vi "Print PDF.vi"(8 "error in (no error)":errorcluster, 11 "PDF Path":path) -> (0 "error out":errorcluster, 2 "Adobe Installed?":bool, 3 "Printed?":bool)   [LabVIEW 2011]
uses:
  <vilib>/registry/registry.llb/Registry RtKey.ctl
  OpenG EXT/file/file.llb/Strip Path Extension - Path__ogtk.vi
  <vilib>/registry/registry.llb/Read Registry Value Simple STR.vi
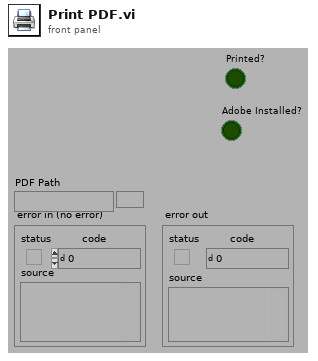
[diagram p1: front panel]
types:
  T1 = typedef "Registry RtKey.ctl" = enum32{"HKEY_CLASSES_ROOT", "HKEY_CURRENT_USER", "HKEY_LOCAL_MACHINE", "HKEY_USERS", "HKEY_PERFORMANCE_DATA", "HKEY_CURRENT_CONFIG", "HKEY_DYN_DATA"}
  T2 = typedef "Registry refnum.ctl" = refnum<k1>
  T3 = cluster{"numSubKeys":i32, "maxSubKeyLen":i32, "maxSubKeyClassLen":i32}
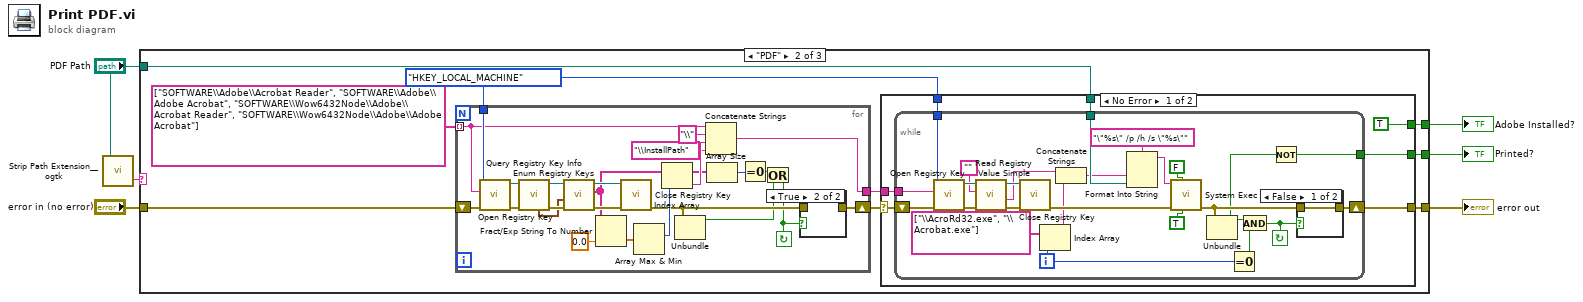
[diagram p0: block diagram]
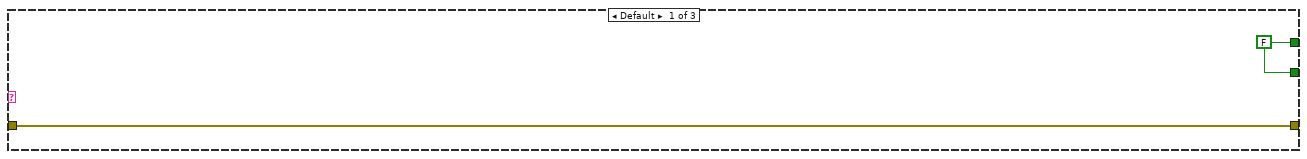
[diagram p2: hidden frame]
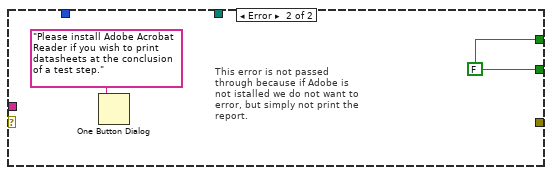
[diagram p5: hidden frame]
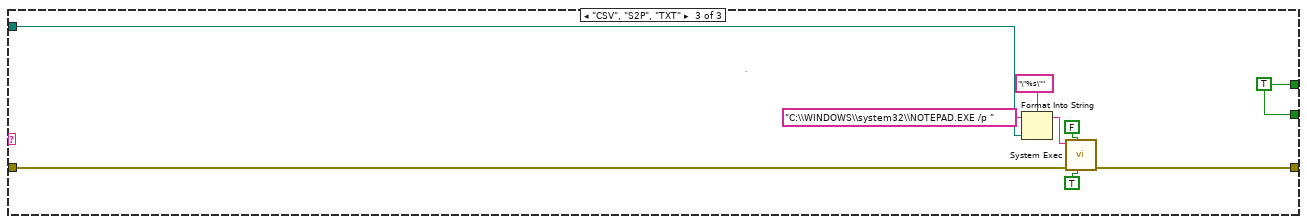
[diagram p6: hidden frame]
diagram:
  n1 = call-poly "Strip Path Extension__ogtk.vi"("path"="PDF Path") -> ("extension"=w1:string)  [unwired: 1 out]
  n2 = case shown="\"PDF\"" w1 {
    tunnel: "error in (no error)" -> [w7 w16 w81]
    tunnel: [w7 w14 w80] -> w5
    tunnel: [w8 w13 w78] -> w4
    tunnel: [w8 w12 w78] -> w3
    tunnel: "PDF Path" -> [_ w11 w86]
    frame Default {
      w8 = FALSE
    }
    frame "PDF" {
      w17 = Registry_RtKey."HKEY_LOCAL_MACHINE" ("root key (HKEY_LOCAL_MACHINE)")
      n3 = for {
        tunnel: [w28] -> w10
        tunnel: w17 -> [w27]
        shift-right: [w24] -> w15
        shift-left: w16 -> [w26]
        tunnel: string[] ["SOFTWARE\\Adobe\\Acrobat Reader", "SOFTWARE\\Adobe\\Adobe Acrobat", "SOFTWARE\\Wow6432Node\\Adobe\\Acrobat Reader", "SOFTWARE\\Wow6432Node\\Adobe\\Adobe Acrobat"] -> [w18] mode=indexing
        stop <- w19 continue-if-true
        n4 = call <vilib>:"Open Registry Key.vi"("error in (no error)"=w26, "subkey"=w18, "root key (HKEY_LOCAL_MACHINE)"=w27) -> ("error out"=w38:errorcluster, "refnum out"=w37:T2)  [unwired: 7 out]
        n5 = call <vilib>:"Query Registry Key Info.vi"("error in (no error)"=w38, "refnum"=w37) -> ("error out"=w40:errorcluster, "refnum out"=w41:T2, "subkey info"=w39:T3)  [unwired: 7 out]
        n6 = call <vilib>:"Enum Registry Keys.vi"("error in (no error)"=w40, "subkey info"=w39, "refnum"=w41) -> ("error out"=w33:errorcluster, "subkeys"=w23:string[], "refnum out"=w32:T2)  [unwired: 6 out]
        n7 = Fract/Exp String To Number(string=w23, default (0 dbl)=0.0) -> (number=w35:dbl[])  [unwired: 3 out]
        n8 = call <vilib>:"Close Registry Key.vi"("error in (no error)"=w33, "refnum"=w32) -> ("error out"=w25:errorcluster)  [unwired: 5 out]
        n9 = Array Max & Min(array=w35) -> (max index (indices)=w34:i32)  [unwired: 3 out]
        n10 = Index Array(array=w23, index=w34) -> (element=w30:string)
        n11 = Unbundle(w25) -> ("status"=w20:bool)  [unwired: 2 out]
        n12 = Concatenate Strings(w18, "\\" ("string"), w30, "\\InstallPath" ("string")) -> (w28:string)
        n13 = Array Size(array=w23) -> (size(s)=w22:i32)
        n14 = Equal To 0?(x=w22) -> (x = 0?=w21:bool)
        n15 = Or(x=w21, y=w20) -> (x .or. y?=w19:bool)
        n16 = case shown="True" w19 {
          tunnel: w25 -> [w42 _]
          tunnel: [w42 _] -> w24
          frame False {
          }
          frame True {
          }
        }
      }
      n17 = case shown="No Error" w15 {
        selector: w15 -> [w45 _]
        tunnel: w11 -> [w49 _]
        tunnel: w10 -> [w48 _]
        tunnel: w17 -> [w47 _]
        tunnel: [w46 _] -> w14
        tunnel: [w44 w77] -> w13
        tunnel: [TRUE w77] -> w12
        frame No Error {
          n18 = while {
            tunnel: w49 -> [w73]
            tunnel: w48 -> [w69]
            tunnel: w47 -> [w68]
            shift-right: [w57] -> w46
            shift-left: w45 -> [w60]
            tunnel: [w54] -> w44
            i -> [w50]
            stop <- w56 continue-if-true
            n19 = call <vilib>:"Open Registry Key.vi"("error in (no error)"=w60, "subkey"=w69, "root key (HKEY_LOCAL_MACHINE)"=w68) -> ("error out"=w67:errorcluster, "refnum out"=w66:T2)  [unwired: 7 out]
            n20 = call-poly <vilib>:"Read Registry Value Simple.vi"("error in (no error)"=w67, "value"="", "refnum"=w66) -> ("error out"=w64:errorcluster, "String/Binary data"=w53:string, "refnum out"=w65:T2)  [unwired: 1 in, 3 out]
            n21 = call <vilib>:"Close Registry Key.vi"("error in (no error)"=w64, "refnum"=w65) -> ("error out"=w62:errorcluster)  [unwired: 5 out]
            n22 = Index Array(array=string[] ["\\AcroRd32.exe", "\\Acrobat.exe"], index=w50) -> (element=w52:string)
            n23 = Concatenate Strings(w53, w52) -> (w61:string)
            n24 = Format Into String(format string="\"%s\" /p /h /s \"%s\"", w61, w73) -> (resulting string=w72:string)  [unwired: 2 in, 1 out]
            n25 = call <vilib>:"System Exec.vi"("run minimized? (F)"=TRUE, "wait until completion? (T)"=FALSE, "error in (no error)"=w62, "command line"=w72) -> ("error out"=w58:errorcluster)  [unwired: 2 in, 5 out]
            n26 = Unbundle(w58) -> ("status"=w55:bool)  [unwired: 2 out]
            n27 = Equal To 0?(x=w50) -> (x = 0?=w59:bool)
            n28 = And(x=w55, y=w59) -> (x .and. y?=w56:bool)
            n29 = Not(x=w55) -> (.not. x?=w54:bool)
            n30 = case shown="False" w56 {
              tunnel: w58 -> [w75 _]
              tunnel: [w75 _] -> w57
              frame False {
              }
              frame True {
              }
            }
          }
        }
        frame Error {
          w77 = FALSE
          # "This error is not passed\nthrough because if Adobe is\nnot istalled we do not want to\nerror, but simply not print the\nreport."
          n31 = One Button Dialog(message="Please install Adobe Acrobat Reader if you wish to print datasheets at the conclusion of a test step." ("string")) -> ()  [unwired: 2 out]
        }
      }
    }
    frame "CSV", "S2P", "TXT" {
      w78 = TRUE
      # "."
      n32 = Format Into String(format string="\"%s\"", initial string="C:\\WINDOWS\\system32\\NOTEPAD.EXE /p " ("format string"), w86) -> (resulting string=w84:string)  [unwired: 1 in, 1 out]
      n33 = call <vilib>:"System Exec.vi"("run minimized? (F)"=TRUE, "wait until completion? (T)"=FALSE, "error in (no error)"=w81, "command line"=w84) -> ("error out"=w80:errorcluster)  [unwired: 2 in, 5 out]
    }
  }
  "error out" <- w5
  "Printed?" <- w4
  "Adobe Installed?" <- w3
